vi "HP81110A Set Arm Source.vi"(8 "error in (no error)":errorcluster, 10 "Arming (Trigger) Source (0:Immediate)":T1(ring), 11 "VISA session":refnum<visa-resource-name>) -> (0 "error out":errorcluster, 3 "dup VISA session":refnum<visa-resource-name>)   [LabVIEW 2009]
doc: "This VI sets the arming (triggering) source. Options are: \n0 = Immediate (internal oscillator)\n1 = Internal PLL\n2 = External \n3 = Manual"
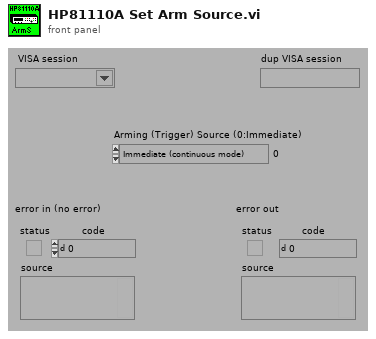
[diagram p1: front panel]
types:
  T1 = enum16{"Immediate (continuous mode)", "Internal PLL", "External", "Manual"}
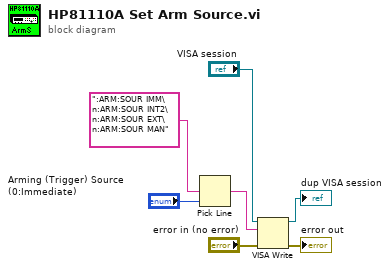
[diagram p0: block diagram]
diagram:
  n1 = Pick Line(multi-line string=":ARM:SOUR IMM\n:ARM:SOUR INT2\n:ARM:SOUR EXT\n:ARM:SOUR MAN", line index="Arming (Trigger) Source (0:Immediate)") -> (output string=w3:string)  [unwired: 1 out]
  n2 = VISA Write(VISA resource name="VISA session", write buffer=w3, error in (no error)="error in (no error)") -> (VISA resource name out=→"dup VISA session":refnum<visa-resource-name>, error out=→"error out":errorcluster)  [unwired: 1 out]
